vi "F Dwf Analog Impedance Comp Reset.vi"(8 "error in (no error)":errorcluster, 11 "hdwf":i32) -> (0 "error out":errorcluster, 3 "function return":i32)   [LabVIEW 2021, in "Olasdwf.lvlib"]
doc: "DWFAPI int FDwfAnalogImpedanceCompReset(HDWF hdwf);"
uses:
  Olasdwf.lvlib
  Windows/System32/dwf.dll
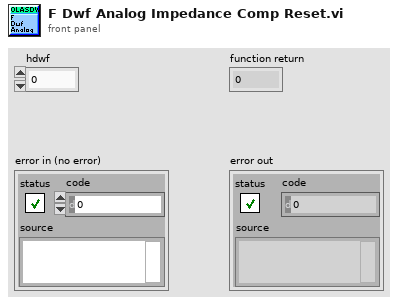
[diagram p1: front panel]
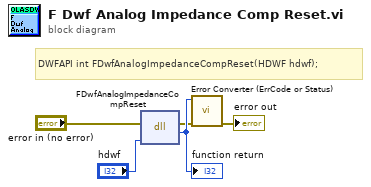
[diagram p0: block diagram]
diagram:
  # "DWFAPI int FDwfAnalogImpedanceCompReset(HDWF hdwf);"
  n1 = dll-call lib="/Windows/System32/dwf.*" fn="FDwfAnalogImpedanceCompReset"(error in="error in (no error)", "hdwf"="hdwf") -> (error out=w2:errorcluster, w5:i32)  [unwired: 3 in, 1 out]
  "function return" <- w5
  n2 = call "Error Converter (ErrCode or Status).vi"("error in (no error)"=w2, "error code"=w5) -> ("error out"=→"error out":errorcluster)  [unwired: 9 in]
